vi "S4GUI.vi"(7 "Tab ObsEng":enum32{"Obs", "CCD modes", "Guider", "Eng"}(tab)) -> ()   [LabVIEW 2018] (continued)
                          }
                          frame "OFF" {
                          }
                          frame "PINHOLE" {
                          }
                          frame "SHUTTER" {
                          }
                        }
                      }
                      frame 3 {
                        n313 = case shown="False" w628 {
                          tunnel: [cluster{u32, u32}[] [{7563008, 7563008}, {7563008, 7563008}] ("Colors [4]") cluster{u32, u32}[] [{16318208, 16318208}, {16318208, 16318208}] ("Colors [4]")] -> w627
                          frame False {
                          }
                          frame True {
                          }
                        }
                        n314 = Not(x=w628) -> (.not. x?=w629:bool)
                      }
                    }
                    "CALW Status" <- w603
                    "PCS" <- w603
                    n315 = property on="CALW Status" class="Bool (strict)"("Colors [4]"=w601) -> ()  [unwired: 2 in, 2 out]
                    n316 = property on="PCS" class="Bool (strict)"("Colors [4]"=w601, "BoolText.Text"=w602) -> ()  [unwired: 2 in, 2 out]
                  }
                  frame #3 {
                    # "ASEL"
                    n317 = Unbundle By Name(w641) -> ("ASEL State"=w640:i32)
                    n318 = Unbundle By Name(w637) -> ("ASEL posname"=w634:string)
                    n319 = local read "ASEL Status"() -> (w635:bool)
                    n320 = case shown="Default" w634 {
                      selector: w634 -> [w642 _ _]
                      tunnel: [w642 "OFF" ("y") "ON" ("y")] -> w633
                      frame Default {
                      }
                      frame "OFF" {
                      }
                      frame "ON" {
                      }
                    }
                    n321 = case shown="3" w640 {
                      tunnel: [cluster{u32, u32}[] [{9868950, 9868950}, {9868950, 9868950}] ("Colors [4]") cluster{u32, u32}[] [{9868950, 9868950}, {9868950, 9868950}] ("Colors [4]") cluster{u32, u32}[] [{16318208, 16318208}, {16318208, 16318208}] ("Colors [4]") cluster{u32, u32}[] [{6618880, 6618880}, {6618880, 6618880}] ("Colors [4]") w660] -> w638
                      tunnel: [FALSE ("WPROT Status") FALSE ("WPROT Status") TRUE FALSE ("WPROT Status") w659] -> w639
                      tunnel: w633 -> [_ _ _ w655 _]
                      tunnel: ["" ("y") "" ("y") "" ("y") w655 "" ("y")] -> w636
                      tunnel: w635 -> [_ _ _ _ w657]
                      frame Default {
                      }
                      frame 0 {
                      }
                      frame 1 {
                      }
                      frame 2 {
                      }
                      frame 3 {
                        n322 = case shown="True" w657 {
                          tunnel: [cluster{u32, u32}[] [{7563008, 7563008}, {7563008, 7563008}] ("Colors [4]") cluster{u32, u32}[] [{16318208, 16318208}, {16318208, 16318208}] ("Colors [4]")] -> w660
                          frame False {
                          }
                          frame True {
                          }
                        }
                        n323 = Not(x=w657) -> (.not. x?=w659:bool)
                      }
                    }
                    "ASEL Status" <- w639
                    "Analyzer" <- w639
                    n324 = property on="Analyzer" class="Bool (strict)"("Colors [4]"=w638, "BoolText.Text"=w636) -> ()  [unwired: 2 in, 2 out]
                    n325 = property on="ASEL Status" class="Bool (strict)"("Colors [4]"=w638) -> ()  [unwired: 2 in, 2 out]
                  }
                  frame #4 {
                    # "GMIR & GFOC"
                    n326 = Unbundle By Name(w670) -> ("GMIR State"=w669:i32, "GFOC State"=w668:i32)
                    n327 = case shown="2" w669 {
                      tunnel: [cluster{u32, u32}[] [{9868950, 9868950}, {9868950, 9868950}] ("Colors [4]") cluster{u32, u32}[] [{9868950, 9868950}, {9868950, 9868950}] ("Colors [4]") cluster{u32, u32}[] [{16318208, 16318208}, {16318208, 16318208}] ("Colors [4]") cluster{u32, u32}[] [{6618880, 6618880}, {6618880, 6618880}] ("Colors [4]") cluster{u32, u32}[] [{16318208, 16318208}, {16318208, 16318208}] ("Colors [4]")] -> w663
                      tunnel: [FALSE ("WPROT Status") FALSE ("WPROT Status") TRUE ("WPROT Status") FALSE ("WPROT Status") TRUE ("WPROT Status")] -> w665
                      frame Default {
                      }
                      frame 0 {
                      }
                      frame 1 {
                      }
                      frame 2 {
                      }
                      frame 3 {
                      }
                    }
                    "GMIR Status" <- w665
                    "GMIR Status 2" <- w665
                    n328 = property on="GMIR Status" class="Bool (strict)"("Colors [4]"=w663) -> ()  [unwired: 2 in, 2 out]
                    n329 = property on="GMIR Status 2" class="Bool (strict)"("Colors [4]"=w663) -> ()  [unwired: 2 in, 2 out]
                    n330 = case shown="Default" w668 {
                      tunnel: [cluster{u32, u32}[] [{9868950, 9868950}, {9868950, 9868950}] ("Colors [4]") cluster{u32, u32}[] [{9868950, 9868950}, {9868950, 9868950}] ("Colors [4]") cluster{u32, u32}[] [{16318208, 16318208}, {16318208, 16318208}] ("Colors [4]") cluster{u32, u32}[] [{6618880, 6618880}, {6618880, 6618880}] ("Colors [4]") cluster{u32, u32}[] [{16318208, 16318208}, {16318208, 16318208}] ("Colors [4]")] -> w664
                      tunnel: [FALSE ("WPROT Status") FALSE ("WPROT Status") TRUE ("WPROT Status") FALSE ("WPROT Status") TRUE ("WPROT Status")] -> w666
                      frame Default {
                      }
                      frame 0 {
                      }
                      frame 1 {
                      }
                      frame 2 {
                      }
                      frame 3 {
                      }
                    }
                    "GFOC Status" <- w666
                    "GFOC Status 2" <- w666
                    n331 = Or(x=w665, y=w666) -> (x .or. y?=w667:bool)
                    n332 = property on="GFOC Status" class="Bool (strict)"("Colors [4]"=w664) -> ()  [unwired: 2 in, 2 out]
                    n333 = property on="GFOC Status 2" class="Bool (strict)"("Colors [4]"=w664) -> ()  [unwired: 2 in, 2 out]
                    n334 = property on="GS led" class="Bool (strict)"("Blinking"=w667, "Value"=w667) -> ()  [unwired: 2 in, 2 out]
                  }
                }
              }
              frame #7 {
                n335 = Unbundle By Name(w693) -> ("Instrument Pos Names"=w692:T21)
                n336 = stacked-sequence {
                  tunnel: w692 -> [w695 w712 w740 w766]
                  tunnel: [_ _ _ w767] -> w691
                  frame #0 {
                    n337 = Unbundle By Name(w695) -> ("WPSEL posname"=w694:string)
                    n338 = case shown="\"L/2\", \"L/4\", \"OFF\"" w694 {
                      selector: w694 -> [_ w696]
                      frame "False", Default {
                      }
                      frame "L/2", "L/4", "OFF" {
                        n339 = First Call?() -> (First Call?: T/F=w697:bool)
                        n340 = case shown="True" w697 {
                          tunnel: w696 -> [_ w698]
                          frame False {
                          }
                          frame True {
                            n341 = case shown="\"False\", Default" w698 {
                              frame "False", Default {
                              }
                              frame "L/2" {
                                w699 = u16 1 items=["OFF", "Lambda/2", "Lambda/4"] ("Lambda Selector")
                                n342 = property on="Lambda Selector" class="Ring (strict)"(error in=errorcluster {"status"=FALSE, "code"=0, "source"=""} ("error in (no error)"), "Value"=w699) -> (error out=w701:errorcluster)  [unwired: 1 in, 1 out]
                                n343 = property on="Lambda Selector" class="Ring (strict)"(error in=w701, "RingText.Text"="Lambda/2" ("Boolean Text.Text")) -> ()  [unwired: 1 in, 2 out]
                              }
                              frame "L/4" {
                                w703 = u16 2 items=["OFF", "Lambda/2", "Lambda/4"] ("Lambda Selector")
                                n344 = property on="Lambda Selector" class="Ring (strict)"(error in=errorcluster {"status"=FALSE, "code"=0, "source"=""} ("error in (no error)"), "Value"=w703) -> (error out=w705:errorcluster)  [unwired: 1 in, 1 out]
                                n345 = property on="Lambda Selector" class="Ring (strict)"(error in=w705, "RingText.Text"="Lambda/4" ("Boolean Text.Text")) -> ()  [unwired: 1 in, 2 out]
                              }
                              frame "OFF" {
                                w708 = u16 0 items=["OFF", "Lambda/2", "Lambda/4"] ("Lambda Selector")
                                (unwired) "Select..." ("Boolean Text.Text")
                                n346 = property on="Lambda Selector" class="Ring (strict)"(error in=errorcluster {"status"=FALSE, "code"=0, "source"=""} ("error in (no error)"), "Value"=w708) -> (error out=w710:errorcluster)  [unwired: 1 in, 1 out]
                                n347 = property on="Lambda Selector" class="Ring (strict)"(error in=w710, "RingText.Text"="OFF" ("Boolean Text.Text")) -> ()  [unwired: 1 in, 2 out]
                              }
                            }
                          }
                        }
                      }
                    }
                  }
                  frame #1 {
                    n348 = Unbundle By Name(w712) -> ("CALW posname"=w711:string)
                    n349 = case shown="\"DEPOLARIZER\", \"OFF\", \"PINHOLE\", \"POLARIZER\", \"SHUTTER\"" w711 {
                      selector: w711 -> [_ w713]
                      frame "False", Default {
                      }
                      frame "DEPOLARIZER", "OFF", "PINHOLE", "POLARIZER", "SHUTTER" {
                        n350 = First Call?() -> (First Call?: T/F=w714:bool)
                        n351 = case shown="True" w714 {
                          tunnel: w713 -> [_ w715]
                          frame False {
                          }
                          frame True {
                            n352 = case shown="\"OFF\"" w715 {
                              frame "False", Default {
                              }
                              frame "POLARIZER" {
                                w716 = u16 1 items=["OFF", "POLARIZER", "PINHOLE", "SHUTTER", "DEPOLARIZER"] ("Calibrator Selector")
                                n353 = property on="Calibrator Selector" class="Ring (strict)"(error in=errorcluster {"status"=FALSE, "code"=0, "source"=""} ("error in (no error)"), "Value"=w716) -> (error out=w718:errorcluster)  [unwired: 1 in, 1 out]
                                n354 = property on="Calibrator Selector" class="Ring (strict)"(error in=w718, "RingText.Text"="POLARIZER" ("Boolean Text.Text")) -> ()  [unwired: 1 in, 2 out]
                              }
                              frame "DEPOLARIZER" {
                                w720 = u16 4 items=["OFF", "POLARIZER", "PINHOLE", "SHUTTER", "DEPOLARIZER"] ("Calibrator Selector")
                                n355 = property on="Calibrator Selector" class="Ring (strict)"(error in=errorcluster {"status"=FALSE, "code"=0, "source"=""} ("error in (no error)"), "Value"=w720) -> (error out=w722:errorcluster)  [unwired: 1 in, 1 out]
                                n356 = property on="Calibrator Selector" class="Ring (strict)"(error in=w722, "RingText.Text"="DEPOLARIZER" ("Boolean Text.Text")) -> ()  [unwired: 1 in, 2 out]
                              }
                              frame "PINHOLE" {
                                w724 = u16 2 items=["OFF", "POLARIZER", "PINHOLE", "SHUTTER", "DEPOLARIZER"] ("Calibrator Selector")
                                n357 = property on="Calibrator Selector" class="Ring (strict)"(error in=errorcluster {"status"=FALSE, "code"=0, "source"=""} ("error in (no error)"), "Value"=w724) -> (error out=w726:errorcluster)  [unwired: 1 in, 1 out]
                                n358 = property on="Calibrator Selector" class="Ring (strict)"(error in=w726, "RingText.Text"="PINHOLE" ("Boolean Text.Text")) -> ()  [unwired: 1 in, 2 out]
                              }
                              frame "SHUTTER" {
                                w728 = u16 3 items=["OFF", "POLARIZER", "PINHOLE", "SHUTTER", "DEPOLARIZER"] ("Calibrator Selector")
                                n359 = property on="Calibrator Selector" class="Ring (strict)"(error in=errorcluster {"status"=FALSE, "code"=0, "source"=""} ("error in (no error)"), "Value"=w728) -> (error out=w730:errorcluster)  [unwired: 1 in, 1 out]
                                n360 = property on="Calibrator Selector" class="Ring (strict)"(error in=w730, "RingText.Text"="SHUTTER" ("Boolean Text.Text")) -> ()  [unwired: 1 in, 2 out]
                              }
                              frame "OFF" {
                                w732 = u16 0 items=["OFF", "POLARIZER", "PINHOLE", "SHUTTER", "DEPOLARIZER"] ("Calibrator Selector")
                                n361 = property on="Calibrator Selector" class="Ring (strict)"(error in=errorcluster {"status"=FALSE, "code"=0, "source"=""} ("error in (no error)"), "Value"=w732) -> (error out=w734:errorcluster)  [unwired: 1 in, 1 out]
                                n362 = property on="Calibrator Selector" class="Ring (strict)"(error in=w734, "RingText.Text"="OFF" ("Boolean Text.Text")) -> ()  [unwired: 1 in, 2 out]
                              }
                            }
                          }
                        }
                      }
                    }
                  }
                  frame #2 {
                    n363 = Unbundle By Name(w740) -> ("WPROT posname"=w736:string)
                    n364 = Concatenate Strings("#Cycles=1  #Exp=1   Waveplate pos=", w736) -> (w738:string)
                    n365 = property on="test msg" class="Str"("Caption.Text"=w738, "Caption.FontBold"=TRUE ("Caption.Font:Bold")) -> ()  [unwired: 2 in, 2 out]
                    n366 = stacked-sequence {
                      tunnel: w736 -> [_ w742]
                      frame #0 {
                        w741 = FALSE
                        "ledP0" <- w741
                        "ledP1" <- w741
                        "ledP2" <- w741
                        "ledP3" <- w741
                        "ledP4" <- w741
                        "ledP5" <- w741
                        "ledP6" <- w741
                        "ledP7" <- w741
                        "ledP8" <- w741
                        "ledP9" <- w741
                        "ledP10" <- w741
                        "ledP11" <- w741
                        "ledP12" <- w741
                        "ledP13" <- w741
                        "ledP14" <- w741
                        "ledP15" <- w741
                      }
                      frame #1 {
                        n367 = case shown="\"WP3\"" w742 {
                          frame Default {
                          }
                          frame "WP1" {
                            n368 = local write "ledP0"(TRUE ("ledP0")) -> ()
                          }
                          frame "WP2" {
                            n369 = local write "ledP1"(TRUE ("ledP0")) -> ()
                          }
                          frame "WP3" {
                            n370 = local write "ledP2"(TRUE ("ledP0")) -> ()
                          }
                          frame "WP4" {
                            n371 = local write "ledP3"(TRUE ("ledP0")) -> ()
                          }
                          frame "WP5" {
                            n372 = local write "ledP4"(TRUE ("ledP0")) -> ()
                          }
                          frame "WP6" {
                            n373 = local write "ledP5"(TRUE ("ledP0")) -> ()
                          }
                          frame "WP7" {
                            n374 = local write "ledP6"(TRUE ("ledP0")) -> ()
                          }
                          frame "WP8" {
                            n375 = local write "ledP7"(TRUE ("ledP0")) -> ()
                          }
                          frame "WP9" {
                            n376 = local write "ledP8"(TRUE ("ledP0")) -> ()
                          }
                          frame "WP10" {
                            n377 = local write "ledP9"(TRUE ("ledP0")) -> ()
                          }
                          frame "WP11" {
                            n378 = local write "ledP10"(TRUE ("ledP0")) -> ()
                          }
                          frame "WP12" {
                            n379 = local write "ledP11"(TRUE ("ledP0")) -> ()
                          }
                          frame "WP13" {
                            n380 = local write "ledP12"(TRUE ("ledP0")) -> ()
                          }
                          frame "WP14" {
                            n381 = local write "ledP13"(TRUE ("ledP0")) -> ()
                          }
                          frame "WP15" {
                            n382 = local write "ledP14"(TRUE ("ledP0")) -> ()
                          }
                          frame "WP16" {
                            n383 = local write "ledP15"(TRUE ("ledP0")) -> ()
                          }
                        }
                      }
                    }
                  }
                  frame #3 {
                    w770 = "OFF" ("Boolean Text.Text")
                    # "Polarimetria:   ASEL = ON  &   (WPSEL =L/2 or L/4)\n\nFotometria:    ASEL=OFF & WPSEL = OFF & CALW = OFF"
                    n384 = Unbundle By Name(w766) -> ("ASEL posname"=w761:string, "WPSEL posname"=w763:string, "CALW posname"=w762:string)
                    n385 = Unbundle By Name(w766) -> ("WPSEL posname"=w773:string, "CALW posname"=w774:string, "ASEL posname"=w768:string)
                    n386 = Equal?(x=w761, y="ON" ("Boolean Text.Text")) -> (x = y?=w764:bool)
                    n387 = case shown="True" w764 {
                      tunnel: w763 -> [w783 w792]
                      tunnel: w762 -> [w782 w786]
                      tunnel: w761 -> [w779 _]
                      tunnel: [FALSE ("Polarimetric Mode") w787] -> w760
                      tunnel: [w775 FALSE ("Photometric Mode")] -> w759
                      frame False {
                        w778 = "OFF" ("Boolean Text.Text")
                        n388 = Equal?(x=w779, y=w778) -> (x = y?=w777:bool)
                        n389 = Equal?(x=w782, y=w778) -> (x = y?=w780:bool)
                        n390 = Equal?(x=w783, y=w778) -> (x = y?=w781:bool)
                        n391 = Compound Arithmetic op=AND(w777, w781, w780) -> (w775:bool)
                      }
                      frame True {
                        n392 = Equal?(x="L/2" ("Boolean Text.Text"), y=w792) -> (x = y?=w793:bool)
                        n393 = Equal?(x="L/4" ("Boolean Text.Text"), y=w792) -> (x = y?=w790:bool)
                        n394 = Not Equal?(x="SHUTTER", y=w786) -> (x != y?=w784:bool)
                        n395 = Or(x=w793, y=w790) -> (x .or. y?=w788:bool)
                        n396 = And(x=w788, y=w784) -> (x .and. y?=w787:bool)
                      }
                    }
                    "Polarimetric Mode" <- w760
                    "Photometric Mode" <- w759
                    n397 = Equal?(x=w770, y=w773) -> (x = y?=w771:bool)
                    n398 = Equal?(x=w770, y=w774) -> (x = y?=w772:bool)
                    n399 = Equal?(x=w770, y=w768) -> (x = y?=w769:bool)
                    n400 = Compound Arithmetic op=AND(w771, w772, w769) -> (invert w767:bool)
                  }
                }
              }
              frame #8 {
                n401 = Unbundle By Name(w799) -> ("ChannelA_Status"=w798:T22, "ChannelB_Status"=w797:T22, "ChannelC_Status"=w795:T22, "ChannelD_Status"=w796:T22)
                n402 = stacked-sequence {
                  tunnel: w798 -> [w887 w943 w995 w1072 _ _ _]
                  tunnel: w797 -> [w886 w941 w994 _ w1093 _ _]
                  tunnel: w796 -> [w884 w938 w992 _ _ _ w1135]
                  tunnel: w795 -> [w885 w939 w993 _ _ w1114 _]
                  frame #0 {
                    n403 = Unbundle By Name(w884) -> ("connection"=w864:bool, "FT"=w846:bool, "Current exp"=w823:dbl, "Cooler ON/OFF"=w878:i16, "Currently temperature"=w875:i16, "Temperature Status"=w872:string, "target  temp"=w808:i16)
                    "Exposure Time ch4" <- w823
                    n404 = Unbundle By Name(w886) -> ("connection"=w866:bool, "FT"=w850:bool, "Current exp"=w834:dbl, "Cooler ON/OFF"=w880:i16, "Currently temperature"=w877:i16, "Temperature Status"=w874:string, "target  temp"=w812:i16)
                    "Exposure Time ch2" <- w834
                    n405 = Unbundle By Name(w887) -> ("connection"=w867:bool, "FT"=w851:bool, "Current exp"=w843:dbl, "Cooler ON/OFF"=w883:i16, "Currently temperature"=w881:i16, "Temperature Status"=w882:string, "target  temp"=w820:i16)
                    "Exposure Time ch1" <- w843
                    n406 = Unbundle By Name(w885) -> ("connection"=w865:bool, "FT"=w848:bool, "Current exp"=w824:dbl, "Cooler ON/OFF"=w879:i16, "Currently temperature"=w876:i16, "Temperature Status"=w873:string, "target  temp"=w809:i16)
                    "Exposure Time ch3" <- w824
                    n407 = Number To Decimal String(number=w808) -> (decimal integer string=→"Target Temp 4":string)  [unwired: 1 in]
                    n408 = Number To Decimal String(number=w809) -> (decimal integer string=→"Target Temp 3":string)  [unwired: 1 in]
                    n409 = Number To Decimal String(number=w812) -> (decimal integer string=→"Target Temp 2":string)  [unwired: 1 in]
                    n410 = Not Equal To 0?(x=w878) -> (x != 0?=w869:bool)
                    n411 = First Call?() -> (First Call?: T/F=w861:bool)
                    n412 = First Call?() -> (First Call?: T/F=w863:bool)
                    n413 = First Call?() -> (First Call?: T/F=w860:bool)
                    n414 = Not Equal To 0?(x=w879) -> (x != 0?=w868:bool)
                    n415 = First Call?() -> (First Call?: T/F=w862:bool)
                    n416 = Number To Decimal String(number=w820) -> (decimal integer string=→"Target Temp 1":string)  [unwired: 1 in]
                    n417 = Number To Fractional String(use system decimal point (T)=FALSE, number=w843, precision (6)=i16 2) -> (F-format string=w840:string)  [unwired: 1 in]
                    n418 = case shown="True" w861 {
                      tunnel: w809 -> [_ w889]
                      frame False {
                      }
                      frame True {
                        n419 = property on="Target Temp 3" class="DigNum (strict)"("Value"=w889) -> ()  [unwired: 2 in, 2 out]
                      }
                    }
                    n420 = case shown="True" w863 {
                      tunnel: w820 -> [_ w891]
                      frame False {
                      }
                      frame True {
                        n421 = property on="Target Temp 1" class="DigNum (strict)"("Value"=w891) -> ()  [unwired: 2 in, 2 out]
                      }
                    }
                    n422 = Number To Fractional String(use system decimal point (T)=FALSE, number=w834, precision (6)=i16 2) -> (F-format string=w835:string)  [unwired: 1 in]
                    n423 = case shown="True" w860 {
                      tunnel: w808 -> [_ w888]
                      frame False {
                      }
                      frame True {
                        n424 = property on="Target Temp 4" class="DigNum (strict)"("Value"=w888) -> ()  [unwired: 2 in, 2 out]
                      }
                    }
                    n425 = Concatenate Strings("Exposure Time ", w840) -> (w839:string)
                    n426 = Number To Fractional String(use system decimal point (T)=FALSE, number=w824, precision (6)=i16 2) -> (F-format string=w825:string)  [unwired: 1 in]
                    n427 = Number To Fractional String(use system decimal point (T)=FALSE, number=w823, precision (6)=i16 2) -> (F-format string=w829:string)  [unwired: 1 in]
                    n428 = Concatenate Strings("Exposure Time ", w835) -> (w833:string)
                    n429 = case shown="True" w862 {
                      tunnel: w812 -> [_ w890]
                      frame False {
                      }
                      frame True {
                        n430 = property on="Target Temp 2" class="DigNum (strict)"("Value"=w890) -> ()  [unwired: 2 in, 2 out]
                      }
                    }
                    n431 = Concatenate Strings("Exposure Time ", w825) -> (w821:string)
                    n432 = Concatenate Strings("Exposure Time ", w829) -> (w822:string)
                    n433 = property on="Exposure Time ch1" class="Slide (strict)"("Caption.Text"=w839) -> ()  [unwired: 2 in, 2 out]
                    n434 = property on="Exposure Time ch2" class="Slide (strict)"("Caption.Text"=w833) -> ()  [unwired: 2 in, 2 out]
                    n435 = property on="Exposure Time ch3" class="Slide (strict)"("Caption.Text"=w821) -> ()  [unwired: 2 in, 2 out]
                    n436 = property on="Exposure Time ch4" class="Slide (strict)"("Caption.Text"=w822) -> ()  [unwired: 2 in, 2 out]
                    n437 = Not Equal To 0?(x=w883) -> (x != 0?=w870:bool)
                    n438 = Not Equal To 0?(x=w880) -> (x != 0?=w871:bool)
                    n439 = case shown="True" w867 {
                      tunnel: w882 -> [_ w922]
                      tunnel: w881 -> [_ w923]
                      tunnel: w870 -> [_ w920]
                      tunnel: [FALSE w920] -> w859
                      tunnel: [i16 0 ("Currently temperature") w923] -> w817
                      tunnel: ["" ("Temperature Status") w922] -> w858
                      tunnel: [FALSE w921] -> w852
                      tunnel: w851 -> [_ w921]
                      frame False {
                      }
                      frame True {
                      }
                    }
                    "Cooler status 1" <- w859
                    "Curr Temp 1" <- w817
                    "Temp Status 1" <- w858
                    "Panel Temp" <- w817
                    "Panel cooler 1" <- w859
                    "FT1" <- w852
                    n440 = case shown="False" w866 {
                      tunnel: w877 -> [_ w914]
                      tunnel: w874 -> [_ w913]
                      tunnel: w871 -> [_ w915]
                      tunnel: [FALSE w915] -> w857
                      tunnel: [i16 0 ("Currently temperature") w914] -> w813
                      tunnel: ["" ("Temperature Status") w913] -> w856
                      tunnel: w850 -> [_ w912]
                      tunnel: [FALSE ("FT") w912] -> w849
                      frame False {
                      }
                      frame True {
                      }
                    }
                    "Panel Temp 2" <- w813
                    "Curr Temp 2" <- w813
                    "Cooler status 2" <- w857
                    "Panel cooler 2" <- w857
                    "Temp Status 2" <- w856
                    "FT2" <- w849
                    n441 = case shown="True" w864 {
                      tunnel: w875 -> [_ w898]
                      tunnel: w872 -> [_ w897]
                      tunnel: w869 -> [_ w899]
                      tunnel: [FALSE w899] -> w854
                      tunnel: [i16 0 ("Currently temperature") w898] -> w801
                      tunnel: ["" ("Temperature Status") w897] -> w853
                      tunnel: w846 -> [_ w896]
                      tunnel: [FALSE ("FT") w896] -> w845
                      frame False {
                      }
                      frame True {
                      }
                    }
                    "Cooler status 4" <- w854
                    "Panel Temp 4" <- w801
                    "Curr Temp 4" <- w801
                    "Temp Status 4" <- w853
                    "Panel cooler 4" <- w854
                    "FT4" <- w845
                    n442 = case shown="True" w865 {
                      tunnel: w876 -> [_ w906]
                      tunnel: w873 -> [_ w905]
                      tunnel: w868 -> [_ w907]
                      tunnel: [FALSE w907] -> w855
                      tunnel: [i16 0 ("Currently temperature") w906] -> w802
                      tunnel: ["" ("Temperature Status") w905] -> w800
                      tunnel: w848 -> [_ w904]
                      tunnel: [FALSE ("FT") w904] -> w847
                      frame False {
                      }
                      frame True {
                      }
                    }
                    "Cooler status 3" <- w855
                    "Panel Temp 3" <- w802
                    "Curr Temp 3" <- w802
                    "Panel cooler 3" <- w855
                    "FT3" <- w847
                    "Temp Status 3" <- w800
                    n443 = Number To Decimal String(number=w813) -> (decimal integer string=w814:string)  [unwired: 1 in]
                    n444 = Number To Decimal String(number=w817) -> (decimal integer string=w818:string)  [unwired: 1 in]
                    n445 = property on="Panel cooler 2" class="Bool (strict)"("BoolText.Text"=w814, "BoolText.Justify"=enum16{"Left", "Center", "Right"}."Right" ("Boolean Text.Justification")) -> ()  [unwired: 2 in, 2 out]
                    n446 = property on="Panel cooler 1" class="Bool (strict)"("BoolText.Text"=w818, "BoolText.Justify"=enum16{"Left", "Center", "Right"}."Right" ("Boolean Text.Justification")) -> ()  [unwired: 2 in, 2 out]
                    n447 = Number To Decimal String(number=w802) -> (decimal integer string=w806:string)  [unwired: 1 in]
                    n448 = Number To Decimal String(number=w801) -> (decimal integer string=w803:string)  [unwired: 1 in]
                    n449 = property on="Panel cooler 3" class="Bool (strict)"("BoolText.Text"=w806, "BoolText.Justify"=enum16{"Left", "Center", "Right"}."Right" ("Boolean Text.Justification")) -> ()  [unwired: 2 in, 2 out]
                    n450 = property on="Panel cooler 4" class="Bool (strict)"("BoolText.Text"=w803, "BoolText.Justify"=enum16{"Left", "Center", "Right"}."Right" ("Boolean Text.Justification")) -> ()  [unwired: 2 in, 2 out]
                  }
                  frame #1 {
                    n451 = Unbundle By Name(w938) -> ("LastFileImage"=→"Last Image ch4":string, "Temperature Status"=w926:string)
                    n452 = Unbundle By Name(w939) -> ("LastFileImage"=→"Last Image ch3":string, "Temperature Status"=w927:string)
                    n453 = Unbundle By Name(w941) -> ("LastFileImage"=→"Last Image ch2":string, "Temperature Status"=w930:string)
                    n454 = Unbundle By Name(w943) -> ("LastFileImage"=→"Last Image ch1":string, "Temperature Status"=w935:string)
                    n455 = case shown="Default" w935 {
                      tunnel: [cluster{u32, u32}[] [{6124107, 6124107}, {6124107, 6124107}] ("Colors [4]") cluster{u32, u32}[] [{6618880, 6618880}, {6618880, 6618880}] ("Colors [4]") cluster{u32, u32}[] [{16318208, 16318208}, {16318208, 16318208}] ("Colors [4]") cluster{u32, u32}[] [{8554752, 8554752}, {8554752, 8554752}] ("Colors [4]")] -> w934
                      tunnel: [FALSE FALSE FALSE TRUE] -> w933
                      frame Default {
                      }
                      frame "TEMPERATURE_STABILIZED" {
                      }
                      frame "TEMPERATURE_NOT_STABILIZED" {
                      }
                      frame "TEMPERATURE_NOT_REACHED" {
                      }
                    }
                    n456 = case shown="\"TEMPERATURE_NOT_REACHED\"" w930 {
                      tunnel: [cluster{u32, u32}[] [{6124107, 6124107}, {6124107, 6124107}] ("Colors [4]") cluster{u32, u32}[] [{6618880, 6618880}, {6618880, 6618880}] ("Colors [4]") cluster{u32, u32}[] [{16318208, 16318208}, {16318208, 16318208}] ("Colors [4]") cluster{u32, u32}[] [{8554752, 8554752}, {8554752, 8554752}] ("Colors [4]")] -> w932
                      tunnel: [FALSE FALSE FALSE TRUE] -> w931
                      frame Default {
                      }
                      frame "TEMPERATURE_STABILIZED" {
                      }
                      frame "TEMPERATURE_NOT_STABILIZED" {
                      }
                      frame "TEMPERATURE_NOT_REACHED" {
                      }
                    }
                    n457 = case shown="\"TEMPERATURE_NOT_REACHED\"" w927 {
                      tunnel: [cluster{u32, u32}[] [{6124107, 6124107}, {6124107, 6124107}] ("Colors [4]") cluster{u32, u32}[] [{6618880, 6618880}, {6618880, 6618880}] ("Colors [4]") cluster{u32, u32}[] [{16318208, 16318208}, {16318208, 16318208}] ("Colors [4]") cluster{u32, u32}[] [{8554752, 8554752}, {8554752, 8554752}] ("Colors [4]")] -> w929
                      tunnel: [FALSE FALSE FALSE TRUE] -> w928
                      frame Default {
                      }
                      frame "TEMPERATURE_STABILIZED" {
                      }
                      frame "TEMPERATURE_NOT_STABILIZED" {
                      }
                      frame "TEMPERATURE_NOT_REACHED" {
                      }
                    }
                    n458 = case shown="\"TEMPERATURE_NOT_REACHED\"" w926 {
                      tunnel: [cluster{u32, u32}[] [{6124107, 6124107}, {6124107, 6124107}] ("Colors [4]") cluster{u32, u32}[] [{6618880, 6618880}, {6618880, 6618880}] ("Colors [4]") cluster{u32, u32}[] [{16318208, 16318208}, {16318208, 16318208}] ("Colors [4]") cluster{u32, u32}[] [{8554752, 8554752}, {8554752, 8554752}] ("Colors [4]")] -> w925
                      tunnel: [FALSE FALSE FALSE TRUE] -> w924
                      frame Default {
                      }
                      frame "TEMPERATURE_STABILIZED" {
                      }
                      frame "TEMPERATURE_NOT_STABILIZED" {
                      }
                      frame "TEMPERATURE_NOT_REACHED" {
                      }
                    }
                    n459 = property on="Cooler status 1" class="Bool (strict)"("Colors [4]"=w934, "Blinking"=w933) -> ()  [unwired: 2 in, 2 out]
                    n460 = property on="Panel cooler 1" class="Bool (strict)"("Colors [4]"=w934, "Blinking"=w933) -> ()  [unwired: 2 in, 2 out]
                    n461 = property on="Cooler status 4" class="Bool (strict)"("Colors [4]"=w925, "Blinking"=w924) -> ()  [unwired: 2 in, 2 out]
                    n462 = property on="Cooler status 3" class="Bool (strict)"("Colors [4]"=w929, "Blinking"=w928) -> ()  [unwired: 2 in, 2 out]
                    n463 = property on="Panel cooler 4" class="Bool (strict)"("Colors [4]"=w925, "Blinking"=w924) -> ()  [unwired: 2 in, 2 out]
                    n464 = property on="Cooler status 2" class="Bool (strict)"("Colors [4]"=w932, "Blinking"=w931) -> ()  [unwired: 2 in, 2 out]
                    n465 = property on="Panel cooler 3" class="Bool (strict)"("Colors [4]"=w929, "Blinking"=w928) -> ()  [unwired: 2 in, 2 out]
                    n466 = property on="Panel cooler 2" class="Bool (strict)"("Colors [4]"=w932, "Blinking"=w931) -> ()  [unwired: 2 in, 2 out]
                  }
                  frame #2 {
                    n467 = Unbundle By Name(w994) -> ("CamStatus"=w987:string, "connection"=w986:bool)
                    n468 = Unbundle By Name(w993) -> ("CamStatus"=w983:string, "connection"=w982:bool)
                    n469 = Unbundle By Name(w992) -> ("CamStatus"=w979:string, "connection"=w978:bool)
                    n470 = Unbundle By Name(w995) -> ("CamStatus"=w991:string, "connection"=w989:bool)
                    n471 = case shown="True" w986 {
                      tunnel: w987 -> [_ w1026]
                      tunnel: [u32 16739417 w1027] -> w984
                      tunnel: ["" ("CamStatus") w1026] -> w985
                      frame False {
                      }
                      frame True {
                        n472 = property on="Acq status string ch2" class="Str"() -> ("Text.BGColor"=w1028:u32)  [unwired: 2 in, 2 out]
                        n473 = case shown="\"\"" w1026 {
                          tunnel: [u32 16688641 w1033 u32 13882323 u32 13882323] -> w1027
                          tunnel: w1028 -> [_ w1032 _ _]
                          frame Default {
                            # "WAITING_EXPOSE_COMMAND"
                          }
                          frame "ACTIVE" {
                            n474 = Equal?(x=w1032, y=u32 16776002) -> (x = y?=w1031:bool)
                            n475 = case shown="False" w1031 {
                              tunnel: [u32 16776002 u32 16449369] -> w1033
                              frame False {
                              }
                              frame True {
                              }
                            }
                          }
                          frame "IDLE" {
                          }
                          frame "" {
                            # "sem resposta do ACS"
                          }
                        }
                      }
                    }
                    "Acq status string ch2" <- w985
                    n476 = case shown="True" w978 {
                      tunnel: w979 -> [_ w998]
                      tunnel: [u32 16739417 w999] -> w976
                      tunnel: ["" ("CamStatus") w998] -> w977
                      frame False {
                      }
                      frame True {
                        n477 = property on="Acq status string ch4" class="Str"() -> ("Text.BGColor"=w1000:u32)  [unwired: 2 in, 2 out]
                        n478 = case shown="\"IDLE\"" w998 {
                          tunnel: [u32 16688641 w1005 u32 13882323 u32 13882323] -> w999
                          tunnel: w1000 -> [_ w1004 _ _]
                          frame Default {
                            # "WAITING_EXPOSE_COMMAND"
                          }
                          frame "ACTIVE" {
                            n479 = Equal?(x=w1004, y=u32 16776002) -> (x = y?=w1003:bool)
                            n480 = case shown="False" w1003 {
                              tunnel: [u32 16776002 u32 16449369] -> w1005
                              frame False {
                              }
                              frame True {
                              }
                            }
                          }
                          frame "IDLE" {
                          }
                          frame "" {
                            # "sem resposta do ACS"
                          }
                        }
                      }
                    }
                    "Acq status string ch4" <- w977
                    n481 = case shown="True" w982 {
                      tunnel: w983 -> [_ w1012]
                      tunnel: [u32 16739417 w1013] -> w980
                      tunnel: ["" ("CamStatus") w1012] -> w981
                      frame False {
                      }
                      frame True {
                        n482 = property on="Acq status string ch3" class="Str"() -> ("Text.BGColor"=w1014:u32)  [unwired: 2 in, 2 out]
                        n483 = case shown="\"\"" w1012 {
                          tunnel: [u32 16688641 w1019 u32 13882323 u32 13882323] -> w1013
                          tunnel: w1014 -> [_ w1018 _ _]
                          frame Default {
                            # "WAITING_EXPOSE_COMMAND"
                          }
                          frame "ACTIVE" {
                            n484 = Equal?(x=w1018, y=u32 16776002) -> (x = y?=w1017:bool)
                            n485 = case shown="False" w1017 {
                              tunnel: [u32 16776002 u32 16449369] -> w1019
                              frame False {
                              }
                              frame True {
                              }
                            }
                          }
                          frame "IDLE" {
                          }
                          frame "" {
                            # "sem resposta do ACS"
                          }
                        }
                      }
                    }
                    "Acq status string ch3" <- w981
                    n486 = case shown="True" w989 {
                      tunnel: w991 -> [_ w1040]
                      tunnel: [u32 16739417 w1041] -> w990
                      tunnel: ["" ("CamStatus") w1040] -> w988
                      frame False {
                      }
                      frame True {
                        n487 = property on="Acq status string ch1" class="Str"() -> ("Text.BGColor"=w1042:u32)  [unwired: 2 in, 2 out]
                        n488 = case shown="\"\"" w1040 {
                          tunnel: [u32 16688641 w1047 u32 13882323 u32 13882323] -> w1041
                          tunnel: w1042 -> [_ w1046 _ _]
                          frame Default {
                            # "WAITING_EXPOSE_COMMAND"
                          }
                          frame "ACTIVE" {
                            n489 = Equal?(x=w1046, y=u32 16776002) -> (x = y?=w1045:bool)
                            n490 = case shown="False" w1045 {
                              tunnel: [u32 16776002 u32 16449369] -> w1047
                              frame False {
                              }
                              frame True {
                              }
                            }
                          }
                          frame "IDLE" {
                          }
                          frame "" {
                            # "sem resposta do ACS"
                          }
                        }
                      }
                    }
                    "Acq status string ch1" <- w988
                    n491 = property on="Acq status string ch2" class="Str"("Text.BGColor"=w984) -> ()  [unwired: 2 in, 2 out]
                    n492 = property on="Acq status string ch1" class="Str"("Text.BGColor"=w990) -> ()  [unwired: 2 in, 2 out]
                    n493 = property on="Acq status string ch3" class="Str"("Text.BGColor"=w980) -> ()  [unwired: 2 in, 2 out]
                    n494 = property on="Acq status string ch4" class="Str"("Text.BGColor"=w976) -> ()  [unwired: 2 in, 2 out]
                  }
                  frame #3 {
                    w1060 = cluster{u32, u32}[] [{16711680, 16711680}, {15400704, 15400704}, {16776722, 0}, {16776722, 0}]  # amarelo
                    w1059 = cluster{u32, u32}[] [{16711680, 16711680}, {6618880, 6618880}, {16776722, 0}, {16776722, 0}]  # verde
                    # "Se ocupacao do disco maior que\n90%, barra em vermelho."
                    # "Atualiza status CANAL 1"
                    n495 = Unbundle By Name(w1072) -> ("Frames done"=w1069:u32, "connection"=→"Channel 1" →"setupCH1":bool, "conf runing"=w1070:bool, "UsedDisk"=w1054:u16, "operational"=w1057:bool)
                    "Exposures Done ch1" <- w1069
                    "Disk Storage ch1" <- w1054
                    n496 = Number To Decimal String(number=w1069) -> (decimal integer string=w1067:string)  [unwired: 1 in]
                    n497 = Greater?(x=w1054, y=u16 90) -> (0:w1064:bool)
                    n498 = Select(t=u32 16711680, s=w1064, f=u32 16860) -> (s? t:f=w1062:u32)
                    n499 = Concatenate Strings("#Exposures Done ", w1067) -> (w1066:string)
                    n500 = Select(t=w1059, s=w1057, f=w1060) -> (s? t:f=w1058:cluster{u32, u32}[])
                    n501 = property on="setupCH1" class="Bool (strict)"("Blinking"=w1070) -> ()  [unwired: 2 in, 2 out]
                    n502 = property on="Exposures Done ch1" class="Slide (strict)"("Caption.Text"=w1066) -> ()  [unwired: 2 in, 2 out]
                    n503 = property on="Channel 1" class="Bool (strict)"("Colors [4]"=w1058) -> ()  [unwired: 2 in, 2 out]
                    n504 = property on="Disk Storage ch1" class="Slide (strict)"("Fill Color"=w1062) -> ()  [unwired: 2 in, 2 out]
                    n505 = Number To Decimal String(number=w1054) -> (decimal integer string=w1055:string)  [unwired: 1 in]
                    n506 = Concatenate Strings("Disk Storage ", w1055, "%" ("string")) -> (w1053:string)
                    n507 = property on="Disk Storage ch1" class="Slide (strict)"("Caption.Text"=w1053) -> ()  [unwired: 2 in, 2 out]
                  }
                  frame #4 {
                    w1081 = cluster{u32, u32}[] [{16711680, 16711680}, {15400704, 15400704}, {16776722, 0}, {16776722, 0}]  # amarelo
                    w1080 = cluster{u32, u32}[] [{16711680, 16711680}, {6618880, 6618880}, {16776722, 0}, {16776722, 0}]  # verde
                    # "Se ocupacao do disco maior que\n90%, barra em vermelho."
                    # "Atualiza status CANAL 2"
                    n508 = Unbundle By Name(w1093) -> ("Frames done"=w1088:u32, "connection"=→"Channel 2" →"setupCH2":bool, "conf runing"=w1091:bool, "UsedDisk"=w1073:u16, "operational"=w1078:bool)
                    "Exposures Done ch2" <- w1088
                    "Disk Storage ch2" <- w1073
                    n509 = Number To Decimal String(number=w1088) -> (decimal integer string=w1089:string)  [unwired: 1 in]
                    n510 = Greater?(x=w1073, y=u16 90) -> (0:w1085:bool)
                    n511 = Select(t=u32 16711680, s=w1085, f=u32 16860) -> (s? t:f=w1082:u32)
                    n512 = Concatenate Strings("#Exposures Done ", w1089) -> (w1087:string)
                    n513 = Select(t=w1080, s=w1078, f=w1081) -> (s? t:f=w1079:cluster{u32, u32}[])
                    n514 = property on="setupCH2" class="Bool (strict)"("Blinking"=w1091) -> ()  [unwired: 2 in, 2 out]
                    n515 = property on="Disk Storage ch2" class="Slide (strict)"("Fill Color"=w1082) -> ()  [unwired: 2 in, 2 out]
                    n516 = property on="Exposures Done ch2" class="Slide (strict)"("Caption.Text"=w1087) -> ()  [unwired: 2 in, 2 out]
                    n517 = property on="Channel 2" class="Bool (strict)"("Colors [4]"=w1079) -> ()  [unwired: 2 in, 2 out]
                    n518 = Number To Decimal String(number=w1073) -> (decimal integer string=w1076:string)  [unwired: 1 in]
                    n519 = Concatenate Strings("Disk Storage ", w1076, "%" ("string")) -> (w1074:string)
                    n520 = property on="Disk Storage ch2" class="Slide (strict)"("Caption.Text"=w1074) -> ()  [unwired: 2 in, 2 out]
                  }
                  frame #5 {
                    w1102 = cluster{u32, u32}[] [{16711680, 16711680}, {15400704, 15400704}, {16776722, 0}, {16776722, 0}]  # amarelo
                    w1101 = cluster{u32, u32}[] [{16711680, 16711680}, {6618880, 6618880}, {16776722, 0}, {16776722, 0}]  # verde
                    # "Se ocupacao do disco maior que\n90%, barra em vermelho."
                    # "Atualiza status CANAL3"
                    n521 = Unbundle By Name(w1114) -> ("Frames done"=w1109:u32, "connection"=→"Channel 3" →"setupCH3":bool, "conf runing"=w1113:bool, "UsedDisk"=w1095:u16, "operational"=w1100:bool)
                    "Exposures Done ch3" <- w1109
                    "Disk Storage ch3" <- w1095
                    n522 = Number To Decimal String(number=w1109) -> (decimal integer string=w1110:string)  [unwired: 1 in]
                    n523 = Greater?(x=w1095, y=u16 90) -> (0:w1106:bool)
                    n524 = Select(t=u32 16711680, s=w1106, f=u32 16860) -> (s? t:f=w1103:u32)
                    n525 = Concatenate Strings("#Exposures Done ", w1110) -> (w1108:string)
                    n526 = property on="setupCH3" class="Bool (strict)"("Blinking"=w1113) -> ()  [unwired: 2 in, 2 out]
                    n527 = property on="Disk Storage ch3" class="Slide (strict)"("Fill Color"=w1103) -> ()  [unwired: 2 in, 2 out]
                    n528 = Select(t=w1101, s=w1100, f=w1102) -> (s? t:f=w1099:cluster{u32, u32}[])
                    n529 = property on="Exposures Done ch3" class="Slide (strict)"("Caption.Text"=w1108) -> ()  [unwired: 2 in, 2 out]
                    n530 = property on="Channel 3" class="Bool (strict)"("Colors [4]"=w1099) -> ()  [unwired: 2 in, 2 out]
                    n531 = Number To Decimal String(number=w1095) -> (decimal integer string=w1097:string)  [unwired: 1 in]
                    n532 = Concatenate Strings("Disk Storage ", w1097, "%" ("string")) -> (w1094:string)
                    n533 = property on="Disk Storage ch3" class="Slide (strict)"("Caption.Text"=w1094) -> ()  [unwired: 2 in, 2 out]
                  }
                  frame #6 {
                    w1123 = cluster{u32, u32}[] [{16711680, 16711680}, {15400704, 15400704}, {16776722, 0}, {16776722, 0}]  # amarelo
                    w1122 = cluster{u32, u32}[] [{16711680, 16711680}, {6618880, 6618880}, {16776722, 0}, {16776722, 0}]  # verde
                    # "Se ocupacao do disco maior que\n90%, barra em vermelho."
                    # "Atualiza status CANAL4"
                    n534 = Unbundle By Name(w1135) -> ("Frames done"=w1130:u32, "connection"=→"Channel 4" →"setupCH4":bool, "conf runing"=w1134:bool, "UsedDisk"=w1116:u16, "operational"=w1120:bool)
                    "Exposures Done ch4" <- w1130
                    "Disk Storage ch4" <- w1116
                    n535 = Number To Decimal String(number=w1130) -> (decimal integer string=w1131:string)  [unwired: 1 in]
                    n536 = Greater?(x=w1116, y=u16 90) -> (0:w1127:bool)
                    n537 = Select(t=u32 16711680, s=w1127, f=u32 16860) -> (s? t:f=w1124:u32)
                    n538 = Concatenate Strings("#Exposures Done ", w1131) -> (w1129:string)
                    n539 = property on="setupCH4" class="Bool (strict)"("Blinking"=w1134) -> ()  [unwired: 2 in, 2 out]
                    n540 = property on="Disk Storage ch4" class="Slide (strict)"("Fill Color"=w1124) -> ()  [unwired: 2 in, 2 out]
                    n541 = Select(t=w1122, s=w1120, f=w1123) -> (s? t:f=w1121:cluster{u32, u32}[])
                    n542 = property on="Exposures Done ch4" class="Slide (strict)"("Caption.Text"=w1129) -> ()  [unwired: 2 in, 2 out]
                    n543 = property on="Channel 4" class="Bool (strict)"("Colors [4]"=w1121) -> ()  [unwired: 2 in, 2 out]
                    n544 = Number To Decimal String(number=w1116) -> (decimal integer string=w1118:string)  [unwired: 1 in]
                    n545 = Concatenate Strings("Disk Storage ", w1118, "%" ("string")) -> (w1115:string)
                    n546 = property on="Disk Storage ch4" class="Slide (strict)"("Caption.Text"=w1115) -> ()  [unwired: 2 in, 2 out]
                  }
                }
              }
              frame #9 {
                n547 = Unbundle By Name(w1142) -> ("Instrument Status.mode"=w1141:bool)
                n548 = case shown="True" w1141 {
                  tunnel: [0 ("t") w1146] -> w1138
                  tunnel: w1142 -> [_ w1145]
                  tunnel: w1136 -> [_ w1144]
                  frame False {
                    # "Fotometria: #PSD = 0"
                  }
                  frame True {
                    n549 = case shown="Default" w1144 {
                      tunnel: [0 ("t") w1159] -> w1146
                      tunnel: w1145 -> [_ w1148]
                      frame 0 {
                        # "Polarimetria em reposuso:  #PSD = 0"
                      }
                      frame Default {
